vi "Calculate Slope Timing.vi"(0 "Current Difference":dbl, 5 "Slew rate A/us":dbl, 7 "Sample Rate":dbl) -> (4 "Slope Record Length":dbl)   [LabVIEW 2020, in "LDO Load Transient_AWG.lvlib"]
uses:
  LDO Load Transient_AWG.lvlib
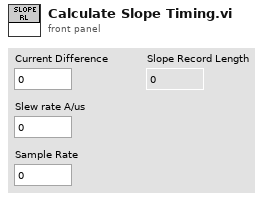
[diagram p1: front panel]
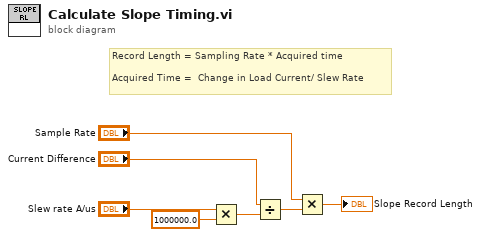
[diagram p0: block diagram]
diagram:
  # "Record Length = Sampling Rate * Acquired time\n\nAcquired Time =  Change in Load Current/ Slew Rate"
  n1 = Multiply(x="Slew rate A/us", y=1000000.0 ("x")) -> (x*y=w1:dbl)
  n2 = Divide(x="Current Difference", y=w1) -> (x/y=w4:dbl)
  n3 = Multiply(x="Sample Rate", y=w4) -> (x*y=→"Slope Record Length":dbl)
